vi "UpdateDatabaseRemote.vi"(3 "Database":T1={"ExperimentDate"=timestamp(3449152219.3203278 s since 1904-01-01), "ImplantDate"=timestamp(3448374613.223979 s since 1904-01-01), "CerebusFolder"="", "Experimenter"="Sara Hanrahan", "NHPName"="Frak", "DeviceType"="USEA", "DeviceSerial"="123456", "DeviceHemisphere"="Right", "DeviceRegion"="Median Nerve", "TaskType"="FingerMove", "TaskComments"="test987", "RecordingComments"="test987", "GeneralObservations"="test987"}, 4 "RecordsSelection":string="\u0000", 5 "CallType":enum16{"Initialize", "Save", "Load"}(ring)) -> (0 "DatabaseOut":T1={"ExperimentDate"=timestamp(3401556199.892892 s since 1904-01-01), "ImplantDate"=timestamp(3401890063 s since 1904-01-01), "CerebusFolder"="", "Experimenter"="Tyler Davis", "NHPName"="201102", "DeviceType"="uECOG", "DeviceSerial"="CG-64BPX-F419", "DeviceHemisphere"="Right", "DeviceRegion"="Hand", "TaskType"="ArmMovementTask.vi", "TaskComments"="", "RecordingComments"="", "GeneralObservations"=""}, 1 "CerebusFoldersDates":string[](array[string])=["20130417-160414", "", "", "", ""], 2 "ExperimentDatesSorted":string[](array[string])=["20130418-120000", "20111015-144319", "20111015-144319", "20111015-144319", "20111015-144319"])   [LabVIEW 2013]
panel:
  # "Do not place ';' or '=' in the comment fields"
  # "Do not place ';' or '=' in the comment fields"
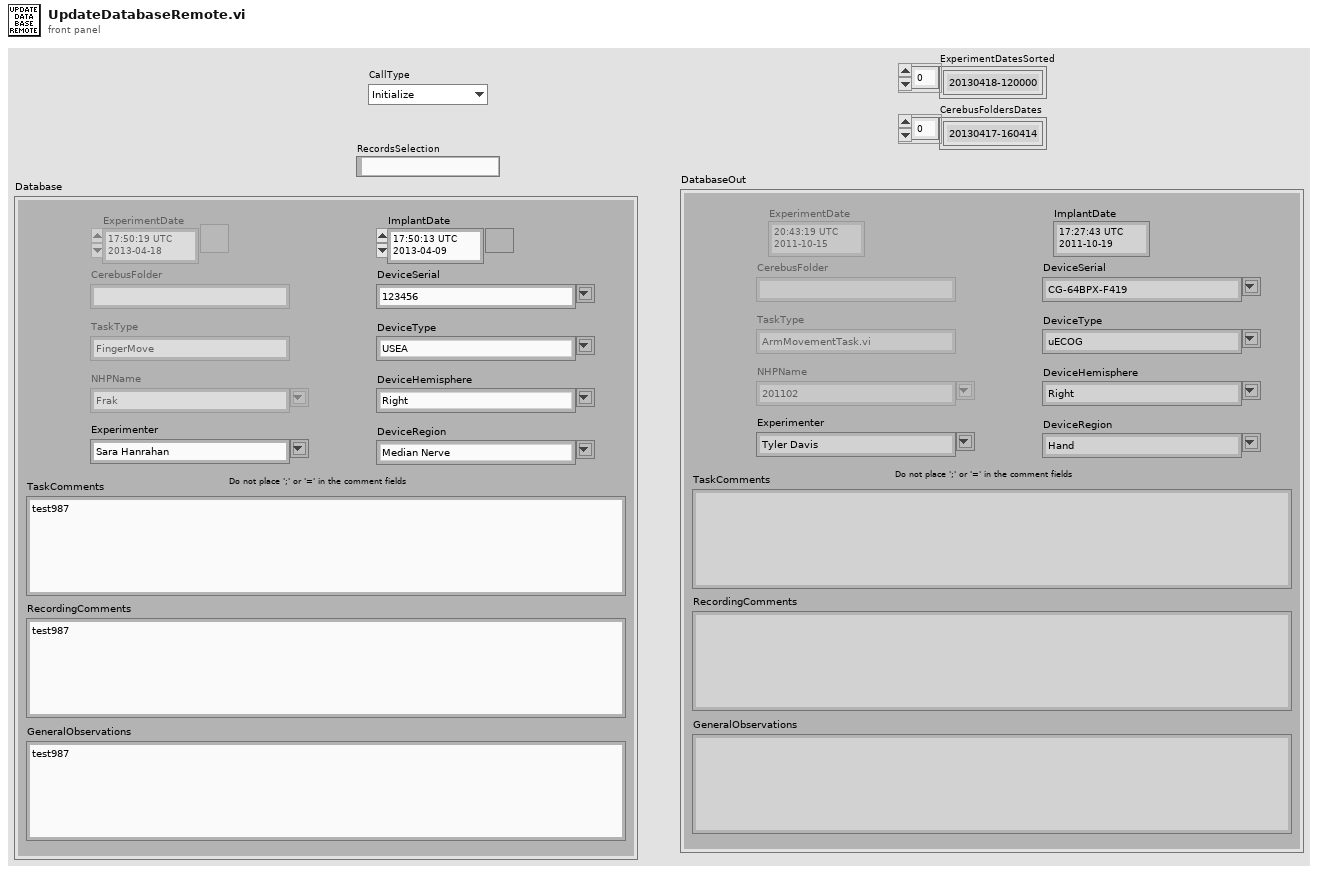
[diagram p1: front panel]
types:
  T1 = cluster{"ExperimentDate":timestamp, "ImplantDate":timestamp, "CerebusFolder":string, "Experimenter":string, "NHPName":string, "DeviceType":string, "DeviceSerial":string, "DeviceHemisphere":string, "DeviceRegion":string, "TaskType":string, "TaskComments":string, "RecordingComments":string, "GeneralObservations":string}
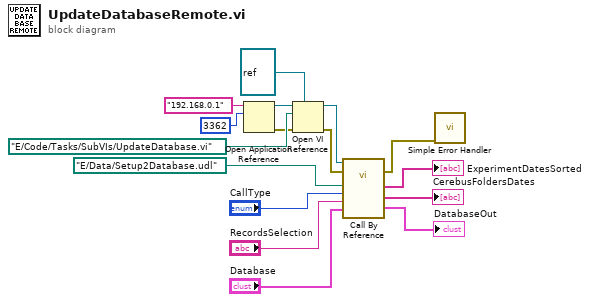
[diagram p0: block diagram]
diagram:
  n1 = Open Application Reference(10:u16 3362 ("port number or service name (3363)"), 11:"192.168.0.1" ("machine name (\"\":  open local reference)")) -> (0:w15:errorcluster, 3:w14:refnum<vi>)  [unwired: 2 in]
  n2 = Open VI Reference(type specifier VI Refnum (for type only)=refnum<vi> refnum, application reference (local)=w14, vi path=path "E:/Code/Tasks/SubVIs/UpdateDatabase.vi", error in (no error)=w15) -> (vi reference=w10:refnum<vi>, error out=w9:errorcluster)  [unwired: 2 in]
  n3 = call-by-ref "?"(reference=w10, error in=w9, "DatabaseIn"="Database", "RecordsSelection"="RecordsSelection", "CallType"="CallType", "DatabaseUDL"=path "E:/Data/Setup2Database.udl") -> (error out=w8:errorcluster, "DatabaseOut"=→"DatabaseOut":T1, "CerebusFoldersDates"=→"CerebusFoldersDates":string[], "ExperimentDatesSorted"=→"ExperimentDatesSorted":string[])  [unwired: 1 out]
  n4 = call <vilib>:"Simple Error Handler.vi"("error in (no error)"=w8) -> ()  [unwired: 4 in, 5 out]
